vi "Acc for animation from modules.vi"(9 "Voltage 3 in":dbl, 10 "Voltage 2 in":dbl, 11 "Voltage 1 in":dbl) -> (1 "Acc 3 out":dbl, 2 "Acc 2 out":dbl, 3 "Acc 1 out":dbl)   [LabVIEW 2020]
doc: "Voltage used in program are large. In case of that it needs to be scaled for usage of animation \nVoltage 1/2/3 in - orginal value of voltage from modules\nAcc 1/2/3 out - the amout of scaled acceleration for proton's animation"
panel:
  # "Important SuBVI - because voltage is large it needs to be scaled"
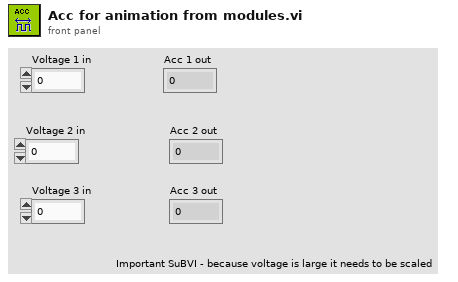
[diagram p1: front panel]
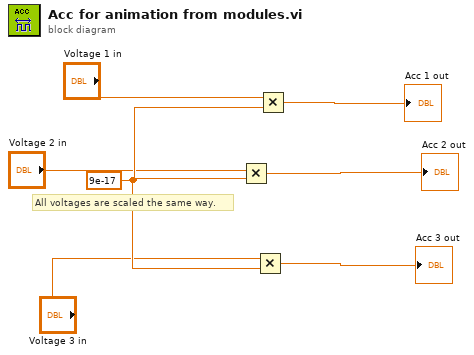
[diagram p0: block diagram]
diagram:
  w7 = 9e-17
  # "All voltages are scaled the same way."
  n1 = Multiply(x="Voltage 2 in", y=w7) -> (x*y=→"Acc 2 out":dbl)
  n2 = Multiply(x="Voltage 3 in", y=w7) -> (x*y=→"Acc 3 out":dbl)
  n3 = Multiply(x="Voltage 1 in", y=w7) -> (x*y=→"Acc 1 out":dbl)
